vi "destroyTelemetry.vi"(8 "error in (no error)":errorcluster, 11 "SAL_Events in":refnum<class "SAL_Events.lvclass">) -> (0 "error out":errorcluster, 3 "SAL_Events out":refnum<class "SAL_Events.lvclass">)   [LabVIEW 2016, in "SAL_Events.lvclass"]
uses:
  SAL_Events.lvclass
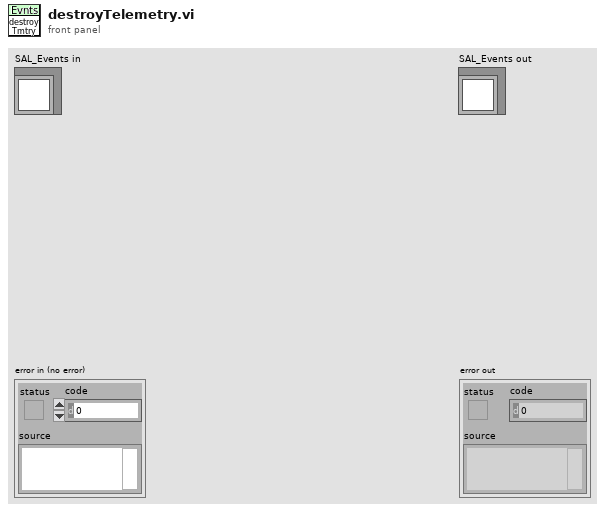
[diagram p1: front panel]
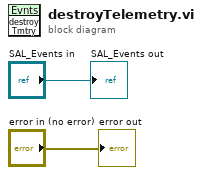
[diagram p0: block diagram]
diagram:
  "error out" <- "error in (no error)"
  "SAL_Events out" <- "SAL_Events in"
